vi "udp_close.vi"(8 "error in":errorcluster, 10 "connection ID":refnum<k16>) -> (0 "error out":errorcluster, 2 "connection ID out":refnum<k16>)   [LabVIEW 2014]
panel:
  # "UDP Close"
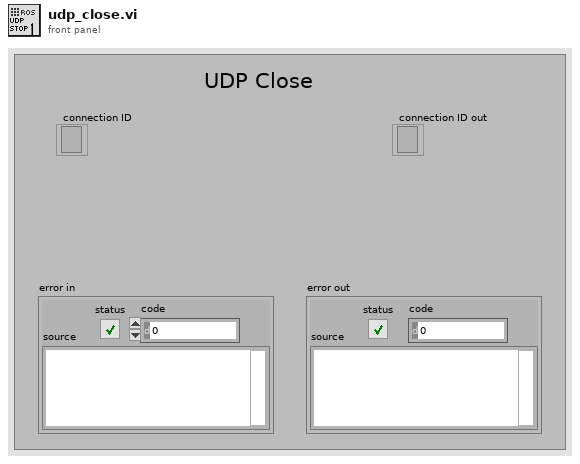
[diagram p1: front panel]
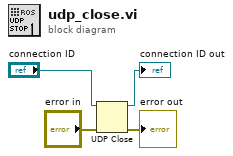
[diagram p0: block diagram]
diagram:
  n1 = UDP Close(connection ID="connection ID", 8:"error in") -> (connection ID out=→"connection ID out":refnum<k16>, error out=→"error out":errorcluster)
